vi "sbRIO Imager.vi"() -> ()   [LabVIEW 2009]
uses:
  <vilib>/real-time/NI_Real-Time Libraries.lvlib
panel:
  in  "target ip address":string
  out "error out":errorcluster
  in  "image file path":path=path "C:/Backup/sbRIO Controller Image/sbrioimg.zip"
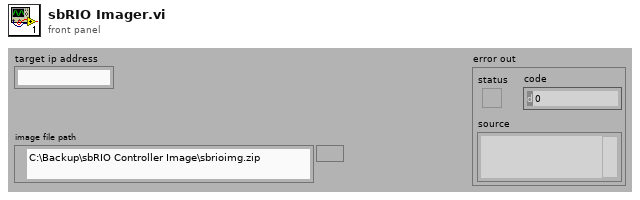
[diagram p1: front panel]
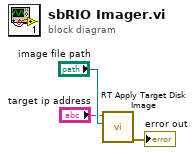
[diagram p0: block diagram]
diagram:
  n1 = call <vilib>:"RT Apply Target Disk Image.vi"("image file path"="image file path", "target address"="target ip address") -> ("error out"=→"error out":errorcluster)  [unwired: 8 in, 1 out]
